vi "PopulateToBooleanRef.vi"(5 "CounterMap":variant, 7 "QDKS Info":T1[](array[typedef]), 8 "error in (no error)":errorcluster, 11 "AllObjs[]":refnum<vi>[](array[refnum])) -> (0 "error out":errorcluster, 3 "AllObjs[] (dup)":refnum<vi>[](array[refnum]))   [LabVIEW 2020, in "NEVSTOP QD Shortcuts.lvlib"]
uses:
  NEVSTOP QD Shortcuts.lvlib
  <resource>/dialog/QuickDrop/QuickDrop QDKS Info.ctl
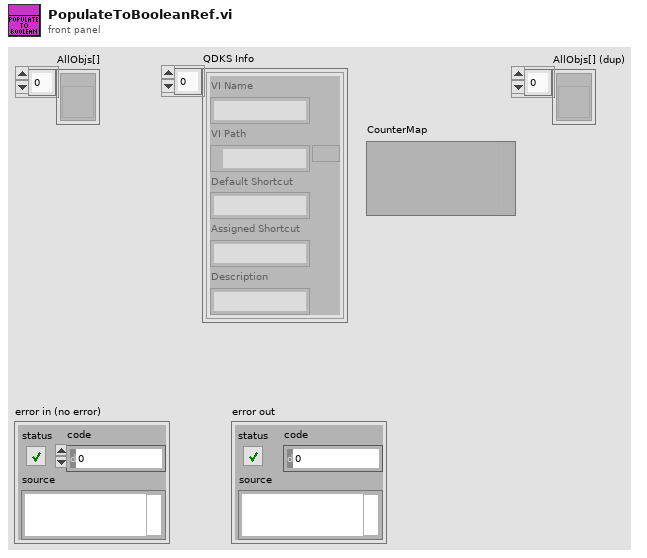
[diagram p1: front panel]
types:
  T1 = typedef "QuickDrop QDKS Info.ctl" = cluster{"VI Name":string, "VI Path":path, "Default Shortcut":string, "Assigned Shortcut":string, "Description":string}
  T2 = typedef "LVFontTypeDef.ctl" = cluster{"Font Name":string, "Size":u16, "Bold":bool, "Italic":bool, "Underline":bool, "Strikeout":bool, "Color":u32}
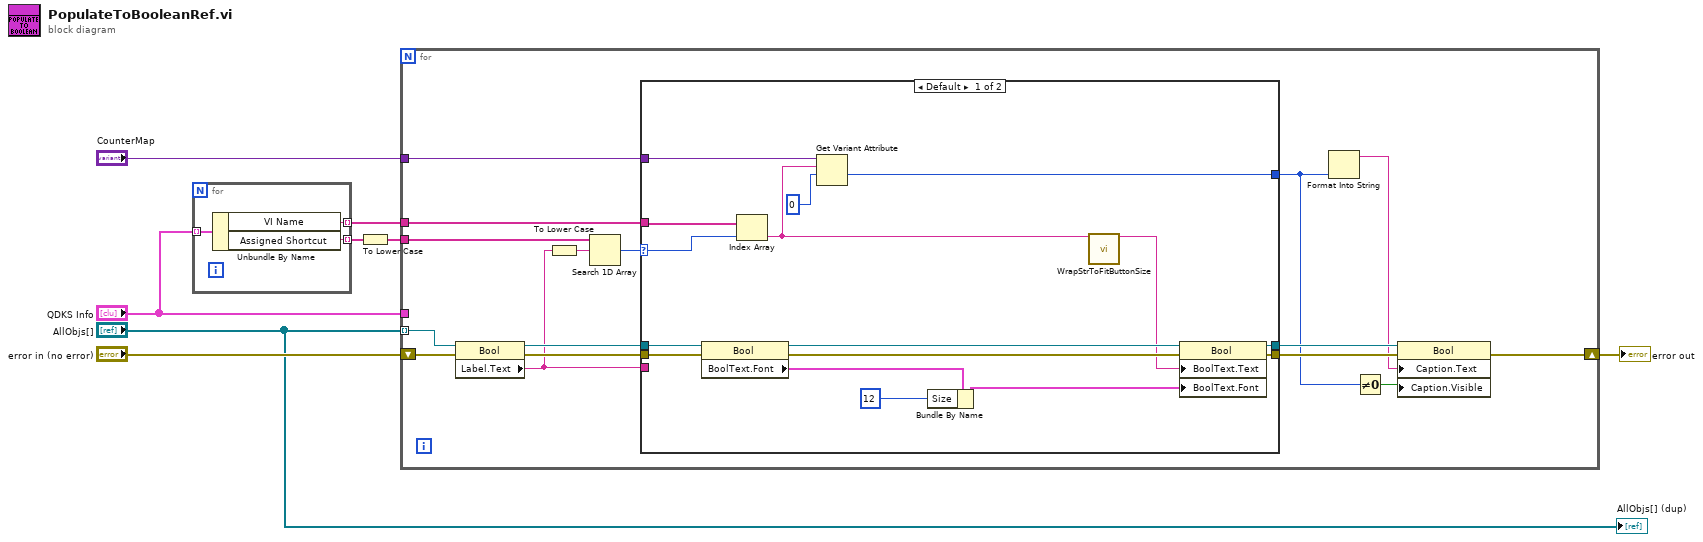
[diagram p0: block diagram]
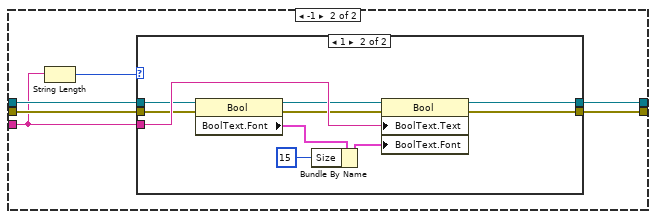
[diagram p2: hidden frame]
diagram:
  n1 = for {
    tunnel: "QDKS Info" -> [w11] mode=indexing
    tunnel: [w10] -> w5 mode=indexing
    tunnel: [w9] -> w4 mode=indexing
    n2 = Unbundle By Name(w11) -> ("VI Name"=w10:string, "Assigned Shortcut"=w9:string)
  }
  n3 = To Lower Case(string=w4) -> (all lower case string=w3:string[])
  n4 = for {
    tunnel: "AllObjs[]" -> [w26] mode=indexing
    tunnel: "QDKS Info" -> [_]
    shift-right: [w15] -> w8
    shift-left: "error in (no error)" -> [w27]
    tunnel: w5 -> [w23]
    tunnel: w3 -> [w25]
    tunnel: "CounterMap" -> [w18]
    n5 = property class="Bool"(reference=w26, error in=w27) -> (reference out=w22:refnum<vi>, error out=w21:errorcluster, "Label.Text"=w19:string)
    n6 = To Lower Case(string=w19) -> (all lower case string=w20:string)
    n7 = Search 1D Array(1D array=w25, element=w20) -> (index of element=w24:i32)  [unwired: 1 in]
    n8 = case shown="Default" w24 {
      selector: w24 -> [w40 _]
      tunnel: w23 -> [w41 _]
      tunnel: w22 -> [w38 w48]
      tunnel: w21 -> [w42 w47]
      tunnel: [w39 w46] -> w17
      tunnel: w19 -> [_ w45]
      tunnel: w18 -> [w33 _]
      tunnel: [w29 w43] -> w16
      tunnel: [w28 _] -> w12
      frame Default {
        n9 = property class="Bool"(reference=w38) -> (reference out=w37:refnum<vi>, "BoolText.Font"=w36:T2)  [unwired: 1 in, 1 out]
        n10 = Index Array(array=w41, index=w40) -> (element=w30:string)
        n11 = Get Variant Attribute(Variant=w33, name=w30, default value (empty Variant)=0) -> (value=w28:i32)  [unwired: 1 in, 3 out]
        n12 = Bundle By Name(cluster=w36, "Size"=u16 12) -> (w35:T2)
        n13 = call "WrapStrToFitButtonSize.vi"("String in"=w30) -> ("Wrapped String"=w31:string)  [unwired: 18 in]
        n14 = property class="Bool"(reference=w37, error in=w42, "BoolText.Text"=w31, "BoolText.Font"=w35) -> (reference out=w29:refnum<vi>, error out=w39:errorcluster)
      }
      frame -1 {
        n15 = String Length(string=w45) -> (length=w44:i32)
        n16 = case shown="1" w44 {
          tunnel: w48 -> [w49 w58]
          tunnel: w47 -> [w50 w56]
          tunnel: [w50 w60] -> w46
          tunnel: w45 -> [_ w59]
          tunnel: [w49 w51] -> w43
          frame Default {
          }
          frame 1 {
            n17 = property class="Bool"(reference=w58, error in=w56) -> (reference out=w57:refnum<vi>, error out=w55:errorcluster, "BoolText.Font"=w54:T2)
            n18 = Bundle By Name(cluster=w54, "Size"=u16 15) -> (w53:T2)
            n19 = property class="Bool"(reference=w57, error in=w55, "BoolText.Text"=w59, "BoolText.Font"=w53) -> (reference out=w51:refnum<vi>, error out=w60:errorcluster)
          }
        }
      }
    }
    n20 = Format Into String(w12) -> (resulting string=w14:string)  [unwired: 3 in, 1 out]
    n21 = Not Equal To 0?(x=w12) -> (x != 0?=w13:bool)
    n22 = property class="Bool"(reference=w16, error in=w17, "Caption.Text"=w14, "Caption.Visible"=w13) -> (error out=w15:errorcluster)  [unwired: 1 out]
  }
  "error out" <- w8
  "AllObjs[] (dup)" <- "AllObjs[]"
